vi "MenuClicked.vi"(8 "error in (no error)":errorcluster, 10 "Full Tag":string, 11 "Menu in":refnum<class "MGI_Menu.lvclass">) -> (0 "error out":errorcluster, 3 "Menu out":refnum<class "MGI_Menu.lvclass">)   [LabVIEW 2016, in "MGI_Menu.lvclass"]
doc: "Simulates the menu click. This will perform an identical action as the user actually clicking the MenuItem.\n\nAuthored by Derek E. Trepanier\nsupport@mooregoodideas.com\nwww.mooregoodideas.com\n\nCopyright (c) 2012, Moore Good Ideas, Inc.\n\nAll rights reserved.\n\nRedistribution and use in source and binary forms, with or without modification, are permitted provided that the following conditions are met:\n\n * Redistributions of source code must retain the above copyright notice, this list of conditions and the following disclaimer.\n * Redistributions in binary form must reproduce the above copyright notice, this list of conditions and the following disclaimer in the documentation and/or other materials provided with the distribution.\n * Neither the name of Moore Good Ideas, Inc. nor the names of its contributors may be used to endorse or promote products derived from this software without specific prior written permission.\n\nTHIS SOFTWARE IS PROVIDED BY THE COPYRIGHT HOLDERS AND CONTRIBUTORS \"AS IS\" AND ANY EXPRESS OR IMPLIED WARRANTIES, INCLUDING, BUT NOT LIMITED TO, THE IMPLIED WARRANTIES OF MERCHANTABILITY AND FITNESS FOR A PARTICULAR PURPOSE ARE DISCLAIMED. IN NO EVENT SHALL THE COPYRIGHT OWNER OR CONTRIBUTORS BE LIABLE FOR ANY DIRECT, INDIRECT, INCIDENTAL, SPECIAL, EXEMPLARY, OR CONSEQUENTIAL DAMAGES (INCLUDING, BUT NOT LIMITED TO, PROCUREMENT OF SUBSTITUTE GOODS OR SERVICES; LOSS OF USE, DATA, OR PROFITS; OR BUSINESS INTERRUPTION) HOWEVER CAUSED AND ON ANY THEORY OF LIABILITY, WHETHER IN CONTRACT, STRICT LIABILITY, OR TORT (INCLUDING NEGLIGENCE OR OTHERWISE) ARISING IN ANY WAY OUT OF THE USE OF THIS SOFTWARE, EVEN IF ADVISED OF THE POSSIBILITY OF SUCH DAMAGE."
uses:
  <userlib>/_MGI/Menu Building/MenuTypes/MGI_Menu.lvclass
  <userlib>/_MGI/Menu Building/MenuTypes/MGI_Menu.lvclass/MGI_Menu.ctl
  <userlib>/_MGI/Menu Building/MenuItem/MGI_MenuItem.lvclass
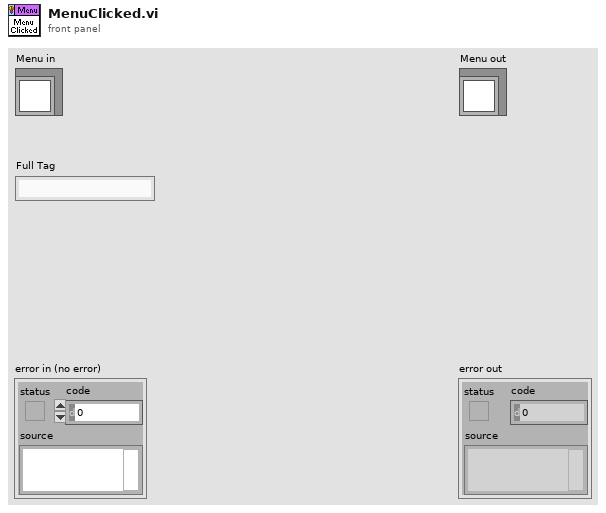
[diagram p1: front panel]
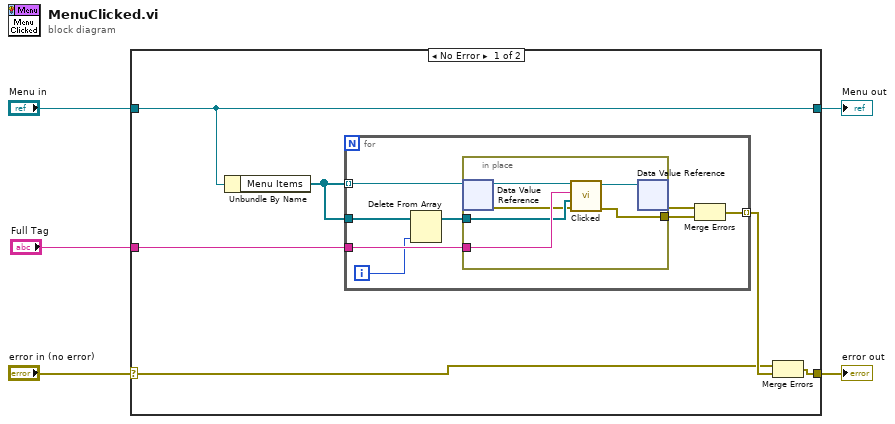
[diagram p0: block diagram]
diagram:
  n1 = case shown="No Error" "error in (no error)" {
    selector: "error in (no error)" -> [w7 w27]
    tunnel: [w10 w27] -> w4
    tunnel: [w11 w26] -> w2
    tunnel: "Menu in" -> [w11 w26]
    tunnel: "Full Tag" -> [w6 _]
    frame No Error {
      n2 = Unbundle By Name(w11) -> ("Menu Items"=w8:refnum<data-value>[])
      n3 = for {
        tunnel: w8 -> [w18] mode=indexing
        tunnel: w6 -> [w19]
        tunnel: [w15] -> w9 mode=indexing
        tunnel: w8 -> [w14]
        i -> [w13]
        n4 = Delete From Array(array=w14, index=w13) -> (array with subset deleted=w12:refnum<data-value>[])  [unwired: 1 in, 1 out]
        n5 = in-place {
          in-place-border: w19 -> [w25]
          in-place-border: [w23] -> w16
          in-place-border: w12 -> [w22]
          n6 = in-place-dvr #1(w18) -> (w21:refnum<class "MGI_MenuItem.lvclass">, w20:errorcluster)
          n7 = call-dynamic "Clicked.vi"("error in (no error)"=w20, "Siblings"=w22, "Clicked Tag"=w25, "MGI_MenuItem in"=w21) -> ("error out"=w23:errorcluster, "MGI_MenuItem out"=w24:refnum<class "MGI_MenuItem.lvclass">)  [unwired: 6 in]
          n8 = in-place-dvr #1(w24) -> (w17:errorcluster)  [unwired: 1 out]
        }
        n9 = Merge Errors(w17, w16) -> (w15:errorcluster)
      }
      n10 = Merge Errors(w7, w9) -> (w10:errorcluster)
    }
    frame Error {
    }
  }
  "error out" <- w4
  "Menu out" <- w2
